vi "Write SODA_.vi"(8 "error in (no error)":errorcluster, 10 "SODA?":bool, 11 "Nestle_Actor in":refnum<class "Nestle_Actor.lvclass">) -> (0 "error out":errorcluster, 3 "Nestle_Actor out":refnum<class "Nestle_Actor.lvclass">)   [LabVIEW 2019, in "Nestle_Actor.lvlib" / "Nestle_Actor.lvclass"]
uses:
  Nestle_Actor.lvclass
  Nestle_Actor.lvclass/Nestle_Actor.ctl
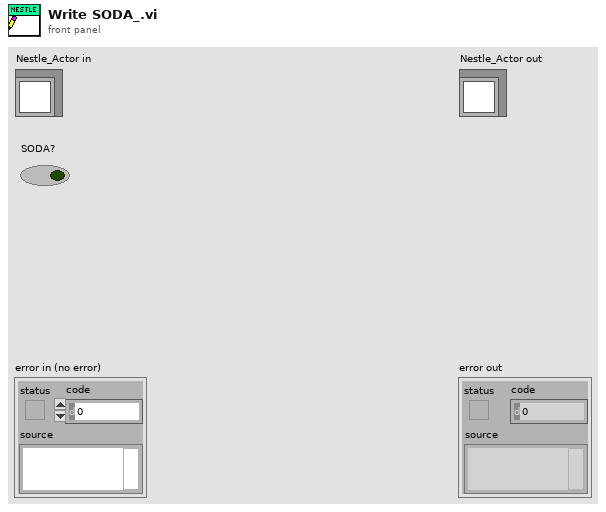
[diagram p1: front panel]
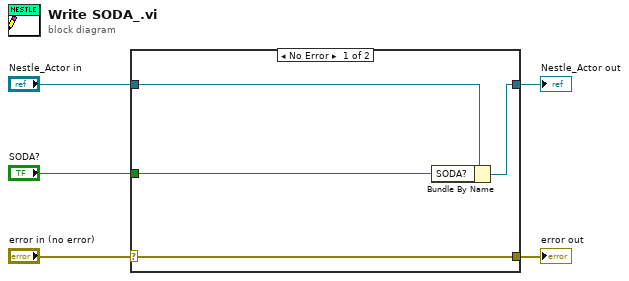
[diagram p0: block diagram]
diagram:
  n1 = case shown="No Error" "error in (no error)" {
    selector: "error in (no error)" -> [w9 w10]
    tunnel: [w9 w10] -> w4
    tunnel: [w7 w11] -> w2
    tunnel: "Nestle_Actor in" -> [w8 w11]
    tunnel: "SODA?" -> [w6 _]
    frame No Error {
      n2 = Bundle By Name(cluster=w8, "SODA?"=w6) -> (w7:refnum<class "Nestle_Actor.lvclass">)
    }
    frame Error {
    }
  }
  "error out" <- w4
  "Nestle_Actor out" <- w2
